vi "Complete Elliptic Integral E.vi"(11 "k":dbl format="%.2f") -> (3 "E(k)":dbl format="%.2f")   [LabVIEW 2014, in "NI_Gmath.lvlib"]
doc: "Computes the Legendre elliptic integral of the second kind. You must manually select the polymorphic instance you want to use."
uses:
  NI_Gmath.lvlib
  lvanlys.dll
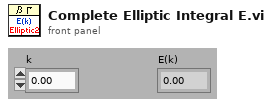
[diagram p1: front panel]
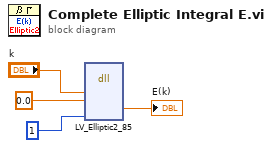
[diagram p0: block diagram]
diagram:
  n1 = dll-call lib="C:/Program Files (x86)/National Instruments/LabVIEW 2014/resource/lvanlys.*" fn="LV_Elliptic2_85"("k"="k", "a"=0.0, "funcType"=1) -> ("Elliptic2(k, a)"=→"E(k)":dbl)  [unwired: 8 in, 2 out]
